vi "ColorDetector-Display.vi"(0 "Upper S&V":u8=255, 1 "Lower S&V":u8=100, 5 "Color 1 Lower":u8=175, 7 "Color 1 Upper":u8=179, 9 "min_Radius":i32=35, 11 "error in (no error)":errorcluster, 12 "max_Radius":i32=60) -> (4 "XYR Found":u32[][](array[numeric]), 15 "error out":errorcluster)   [LabVIEW 2014, in "QwaveSys RPi Training Library.lvlib"]
uses:
  <vilib>/Q-Wave Systems/QwaveSys RPi Training Package (Demo)/Addons/QwaveSys RPi Training Library.lvlib
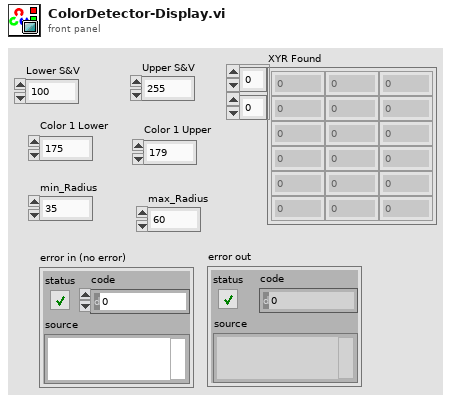
[diagram p1: front panel]
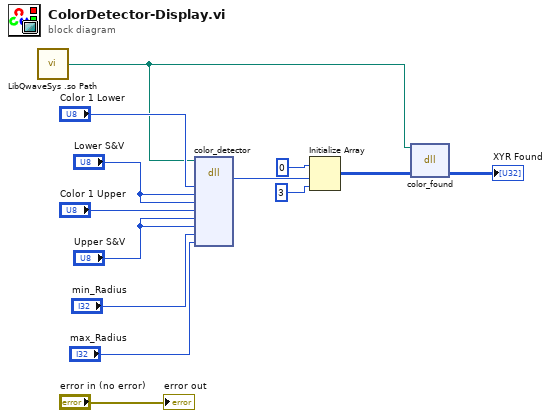
[diagram p0: block diagram]
diagram:
  n1 = call <vilib>:"LibQwaveSys .so Path.vi"() -> ("Lib QwaveSys .so Path"=w1:path)  [unwired: 5 in]
  n2 = dll-call lib="libqwavesys.so" fn="color_detector"(path in=w1, "lower_h"="Color 1 Lower", "lower_s"="Lower S&V", "lower_v"="Lower S&V", "upper_h"="Color 1 Upper", "upper_s"="Upper S&V", "upper_v"="Upper S&V", "min_radius"="min_Radius", "max_radius"="max_Radius") -> ("return type"=w3:i32)  [unwired: 10 in, 2 out]
  n3 = Initialize Array "Initialize Array"(u32 0 ("element"), w3, 3 ("dimension size")) -> (w4:u32[][])
  n4 = dll-call lib="libqwavesys.so" fn="color_found"(path in=w1, "found"=w4) -> ("found"=→"XYR Found":u32[][])  [unwired: 3 in, 2 out]
  "error out" <- "error in (no error)"
